vi "Error_2.vi"(7 "Current PNG Filename":string, 8 "error in (no error)":errorcluster, 11 "Folder Path":path) -> (0 "error out":errorcluster)   [LabVIEW 2023]
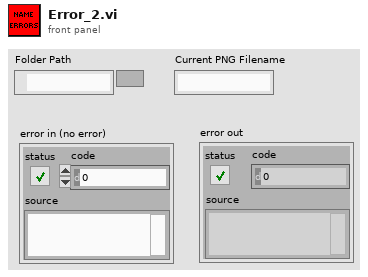
[diagram p1: front panel]
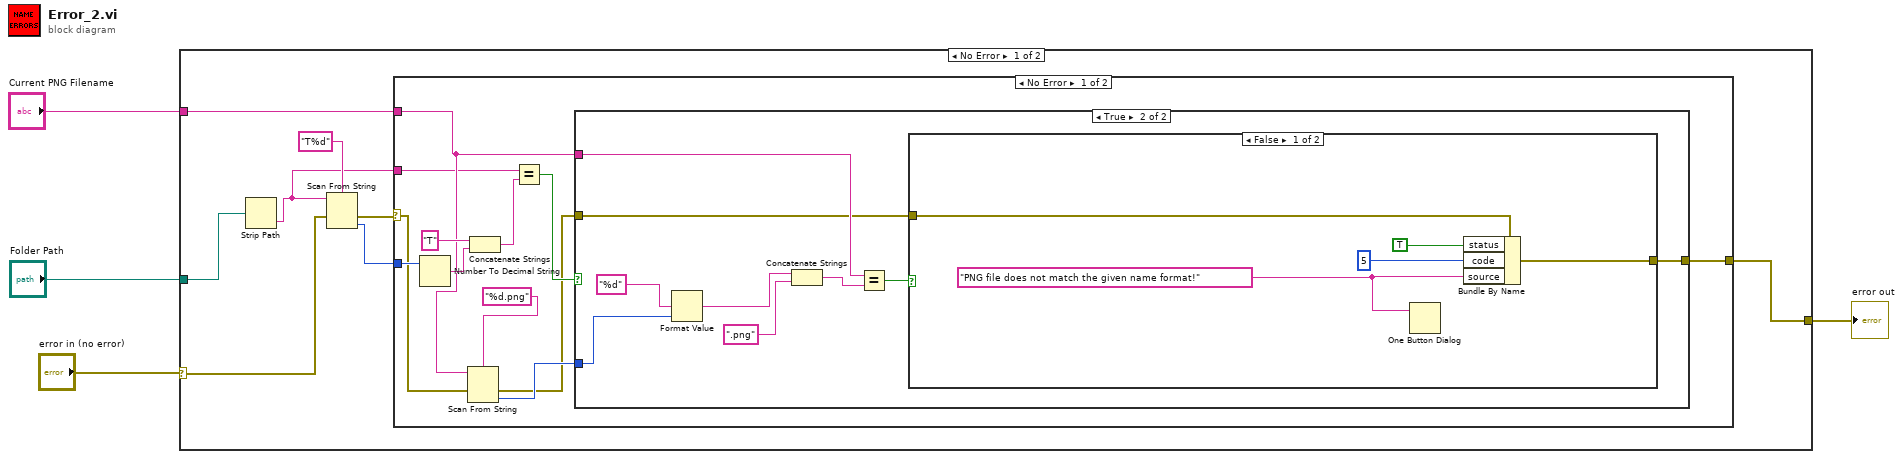
[diagram p0: block diagram]
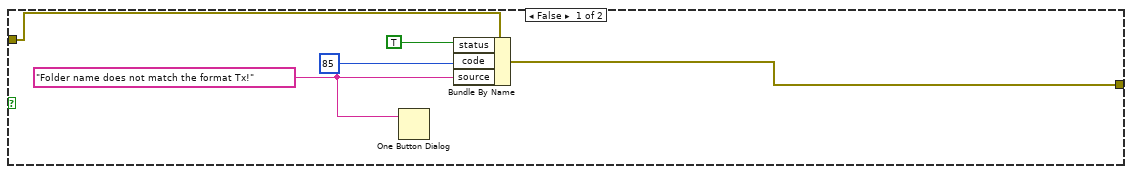
[diagram p2: hidden frame]
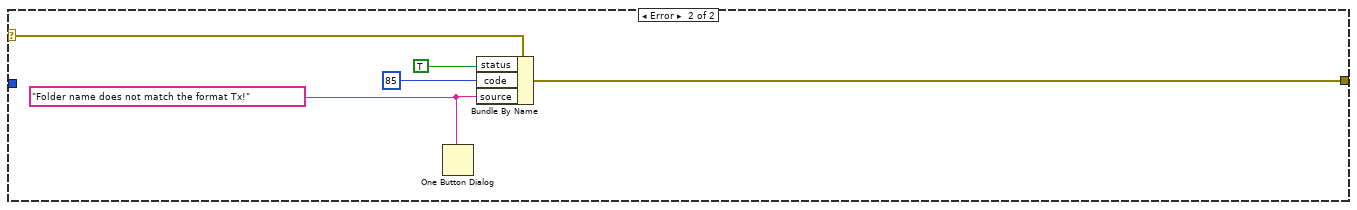
[diagram p4: hidden frame]
diagram:
  n1 = case shown="No Error" "error in (no error)" {
    selector: "error in (no error)" -> [w10 w50]
    tunnel: "Current PNG Filename" -> [w8 _]
    tunnel: "Folder Path" -> [w12 _]
    tunnel: [w6 w50] -> w1
    frame No Error {
      n2 = Strip Path(path=w12) -> (name=w5:string)  [unwired: 1 out]
      n3 = Scan From String(format string="T%d", input string=w5, error in=w10) -> (error out=w9:errorcluster, output 1=w7:i32)  [unwired: 2 in, 2 out]
      n4 = case shown="No Error" w9 {
        selector: w9 -> [w15 w49]
        tunnel: w8 -> [w17 _]
        tunnel: w5 -> [w13 _]
        tunnel: w7 -> [w24 _]
        tunnel: [w19 w46] -> w6
        frame No Error {
          n5 = Number To Decimal String(number=w24) -> (decimal integer string=w23:string)  [unwired: 1 in]
          n6 = Scan From String(format string="%d.png", input string=w17, error in=w15) -> (error out=w14:errorcluster, output 1=w16:i32)  [unwired: 2 in, 2 out]
          n7 = Concatenate Strings("T", w23) -> (w21:string)
          n8 = Equal?(x=w13, y=w21) -> (x = y?=w20:bool)
          n9 = case shown="True" w20 {
            tunnel: w14 -> [w29 w33]
            tunnel: w17 -> [_ w35]
            tunnel: [w25 w32] -> w19
            tunnel: w16 -> [_ w30]
            frame False {
              w26 = "Folder name does not match the format Tx!"
              n10 = One Button Dialog(message=w26) -> ()  [unwired: 1 in, 1 out]
              n11 = Bundle By Name(cluster=w29, "status"=TRUE, "code"=85, "source"=w26) -> (w25:errorcluster)
            }
            frame True {
              n12 = Format Value(format string="%d", value (0)=w30) -> (output string=w31:string)  [unwired: 1 in]
              n13 = Concatenate Strings(w31, ".png") -> (w36:string)
              n14 = Equal?(x=w35, y=w36) -> (x = y?=w34:bool)
              n15 = case shown="False" w34 {
                tunnel: w33 -> [w43 w44]
                tunnel: [w42 w44] -> w32
                frame False {
                  w39 = "PNG file does not match the given name format!"
                  n16 = One Button Dialog(message=w39) -> ()  [unwired: 1 in, 1 out]
                  n17 = Bundle By Name(cluster=w43, "status"=TRUE, "code"=5, "source"=w39) -> (w42:errorcluster)
                }
                frame True {
                }
              }
            }
          }
        }
        frame Error {
          w47 = "Folder name does not match the format Tx!"
          n18 = One Button Dialog(message=w47) -> ()  [unwired: 1 in, 1 out]
          n19 = Bundle By Name(cluster=w49, "status"=TRUE, "code"=85, "source"=w47) -> (w46:errorcluster)
        }
      }
    }
    frame Error {
    }
  }
  "error out" <- w1
